vi "Finalize To Settings.vi"(8 "error in":errorcluster, 11 "RDMA Rx Transfer Configuration in":refnum<class "RDMA Transfer Rx Configuration.lvclass">) -> (0 "error out":errorcluster, 2 "settings":cluster{"key":string, "value":string}[](array[cluster]), 3 "RDMA Rx Transfer Configuration out":refnum<class "RDMA Transfer Rx Configuration.lvclass">)   [LabVIEW 2020, in "RDMA.lvlib" / "RDMA Transfer Rx Configuration.lvclass"]
uses:
  RDMA Transfer Rx Configuration.lvclass
  RDMA Transfer Rx Configuration.lvclass/RDMA Transfer Rx Configuration.ctl
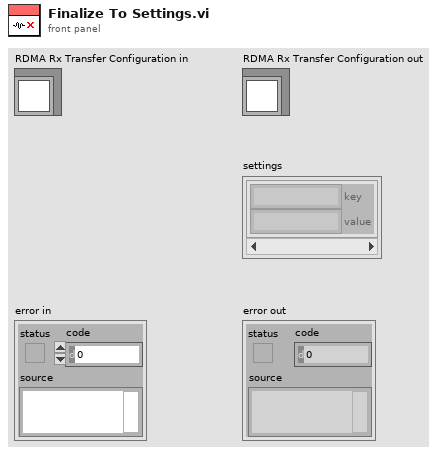
[diagram p1: front panel]
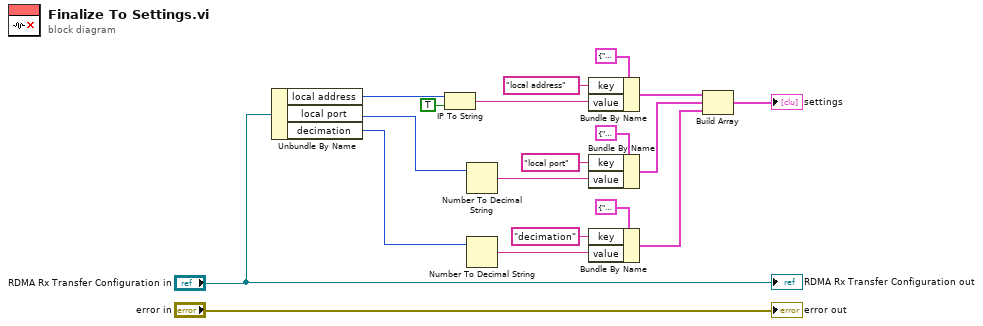
[diagram p0: block diagram]
diagram:
  n1 = Unbundle By Name("RDMA Rx Transfer Configuration in") -> ("local address"=w15:u32, "local port"=w10:u16, "decimation"=w2:u16)
  n2 = IP To String(1:TRUE ("dot notation? (F)"), 2:w15) -> (0:w13:string)
  n3 = Number To Decimal String(number=w10) -> (decimal integer string=w9:string)  [unwired: 1 in]
  n4 = Number To Decimal String(number=w2) -> (decimal integer string=w3:string)  [unwired: 1 in]
  n5 = Bundle By Name(cluster=cluster{"key":string, "value":string} {"key"="", "value"=""} ("setting"), "key"="local address", "value"=w13) -> (w8:cluster{"key":string, "value":string})
  n6 = Bundle By Name(cluster=cluster{"key":string, "value":string} {"key"="", "value"=""} ("setting"), "key"="local port", "value"=w9) -> (w7:cluster{"key":string, "value":string})
  n7 = Bundle By Name(cluster=cluster{"key":string, "value":string} {"key"="", "value"=""} ("setting"), "key"="decimation", "value"=w3) -> (w1:cluster{"key":string, "value":string})
  n8 = Build Array(w8, w7, w1) -> (→"settings":cluster{"key":string, "value":string}[])
  "error out" <- "error in"
  "RDMA Rx Transfer Configuration out" <- "RDMA Rx Transfer Configuration in"
